vi "Sort 3 Numbers (SubVI).vi"(11 "Array In":u16[](array[numeric])=[0, 0, 0]) -> (3 "Array Out":u16[](array[numeric]))   [LabVIEW 2015]
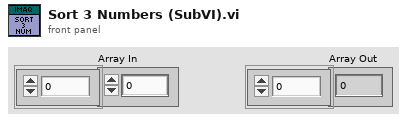
[diagram p1: front panel]
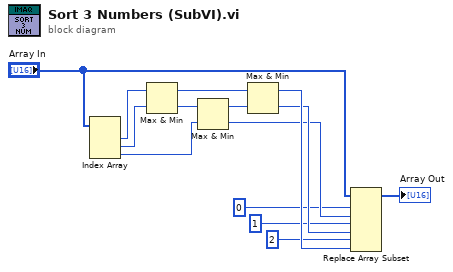
[diagram p0: block diagram]
diagram:
  n1 = Index Array(array="Array In") -> (element #1=w1:u16, element #2=w2:u16, element #3=w4:u16)  [unwired: 3 in]
  n2 = Max & Min(x=w1, y=w2) -> (max(x,y)=w6:u16, min(x,y)=w3:u16)
  n3 = Max & Min(x=w3, y=w4) -> (max(x,y)=w5:u16, min(x,y)=w10:u16)
  n4 = Max & Min(x=w6, y=w5) -> (max(x,y)=w12:u16, min(x,y)=w11:u16)
  n5 = Replace Array Subset(array="Array In", new element #1=w10, index #1=0 ("index"), new element #2=w11, index #2=1 ("index"), new element #3=w12, index #3=2 ("index")) -> (→"Array Out":u16[])
